vi "DS360 Set amplitude.vi"(8 "error in (no error)":T1, 10 "Amplitude (p-p) (0)":dbl, 11 "GPIB address":string) -> (0 "error out":T1, 3 "address out":string)   [LabVIEW 2025, in "MyDS360.lvlib"]
uses:
  MyDS360.lvlib
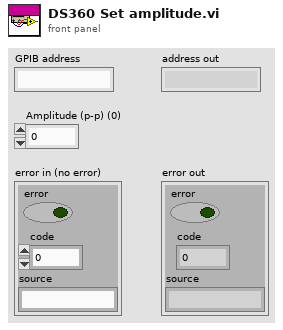
[diagram p1: front panel]
types:
  T1 = cluster{"error":bool, "code":i32, "source":string}
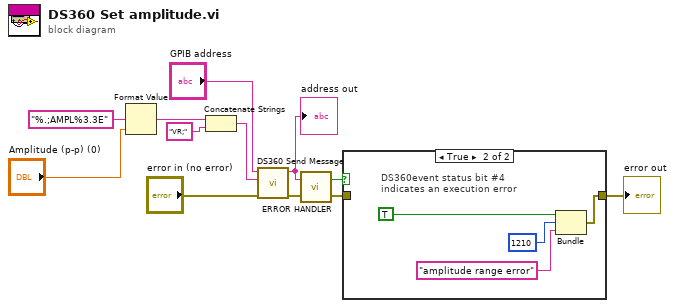
[diagram p0: block diagram]
diagram:
  n1 = Format Value(format string="%.;AMPL%3.3E", value (0)="Amplitude (p-p) (0)") -> (output string=w3:string)  [unwired: 1 in]
  n2 = Concatenate Strings(w3, "VR;") -> (w1:string)
  n3 = call "DS360 Send Message.vi"("address string"="GPIB address", "write buffer"=w1, "error in"="error in (no error)") -> ("address out"=w8:string, "error out"=w9:T1)  [unwired: 3 in, 2 out]
  "address out" <- w8
  n4 = call "ERROR HANDLER.vi"("error in"=w9, "GPIB address"=w8) -> ("error out"=w10:T1, "error found"=w11:bool)
  n5 = case shown="True" w11 {
    tunnel: w10 -> [w13 _]
    tunnel: [w13 w14] -> w12
    frame False {
    }
    frame True {
      # "DS360event status bit #4\nindicates an execution error"
      n6 = Bundle(TRUE, 1210, "amplitude range error") -> (w14:errorcluster)  [unwired: 1 in]
    }
  }
  "error out" <- w12
